vi "Barcode test.vi"() -> ()   [LabVIEW 2019]
uses:
  LLB/Commonly VI/Main Glb.vi
  LLB/Commonly VI.lvlib
  Ctrl/MeasureDisplayTab.ctl
panel:
  in  "AddTable for S2":string[][](table)=[["PCBA BARCODE", ""], ["硬體(Tool初始化)", ""], ["company(Tool初始化)", ""], ["耗電流 uA(電流表)", "T"], ["電池負載電壓", "T"], ["晶片ID(Tool FORMAT)", "F"], ["雷雕ID(TOOl scan、藍芽接收器)", "S"], ["Format(Tool FORMAT)", "F"], ["Programe(Tool Programe)", "P"]]
  out "output array":string[][](array[string])
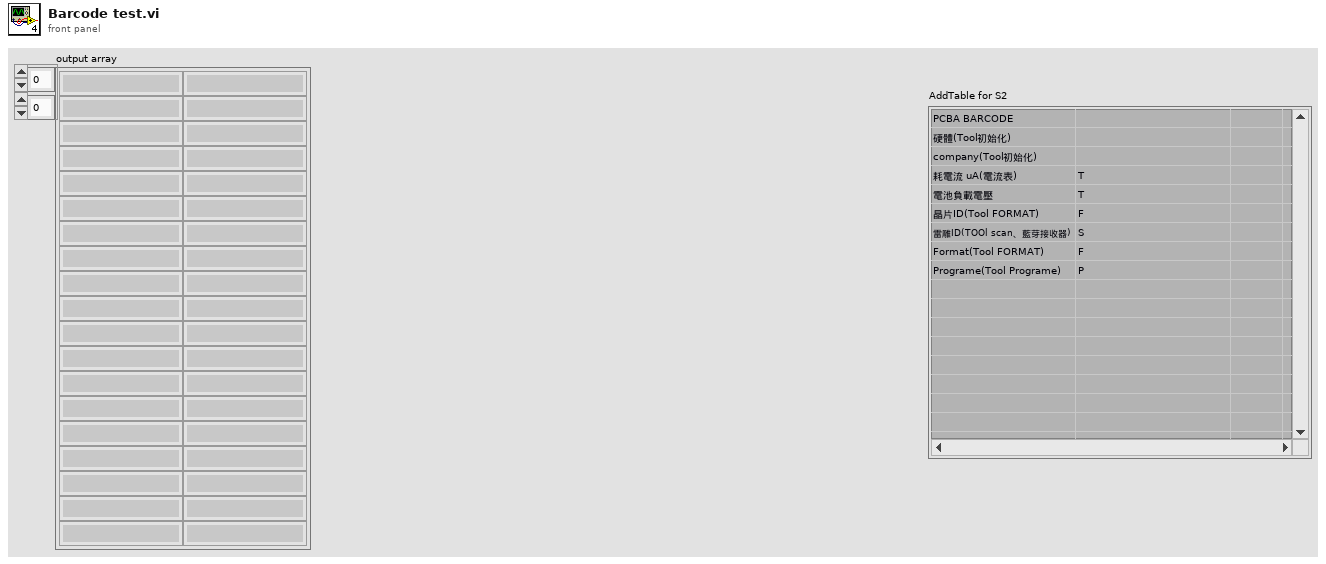
[diagram p1: front panel]
types:
  T1 = enum16{"initial", "Add", "Write", "Replace", "Delete", "REad"}
  T2 = typedef "MeasureDisplayTab.ctl" = enum16{"Tray Barcode", "PCBA BARCODE", "硬體(Tool初始化)", "company(Tool初始化)", "耗電流 uA(電流表)", "電池負載電壓", "晶片ID(Tool FORMAT)", "雷雕ID(TOOl scan、藍芽接收器)", "Format(Tool FORMAT)", "Programe(Tool Programe)", "MAC(藍芽接收器)", "ID(藍芽接收器)", "KPA(藍芽接收器)", "溫度(藍芽接收器)", "SENSOR電池電壓(藍芽接收器)", "RSSI(藍芽接收器)", "SensorType_315(FSK scan)", "FSKsnVol_315(FSK scan)", "FSKscanl_315(FSK scan)", "P_315(FSK scan)", "T_315(FSK scan)", "SensorType_433(ASK scan)", "ASKsnVol_433(ASK scan)", "ASKscan_433(ASK scan)", "P_433(ASK scan)", "T_433(ASK scan)", "測高Data"}
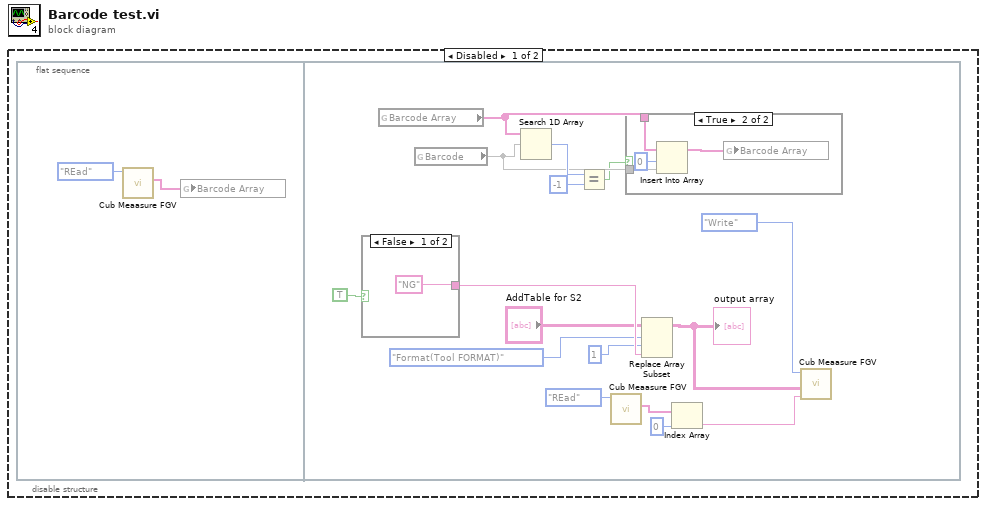
[diagram p0: block diagram]
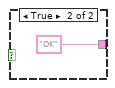
[diagram p2: hidden frame]
diagram:
  n1 = disable-structure shown="Disabled" {
    frame Disabled {
      n2 = flat-sequence {
        frame #0 {
          n3 = call "Cub Meaasure FGV.vi"("Enum"=T1."REad") -> ("Barcode Array"=w1:string[])  [unwired: 9 in, 1 out]
          n4 = global write "Main Glb.vi" "Barcode Array"(w1) -> ()
        }
        frame #1 {
          n5 = case shown="False" TRUE {
            tunnel: ["NG" "OK"] -> w7
            frame False {
            }
            frame True {
            }
          }
          n6 = global read "Main Glb.vi" "Barcode Array"() -> (w16:string[])
          n7 = global read "Main Glb.vi" "Barcode"() -> (w15)
          n8 = Search 1D Array(1D array=w16, element=w15) -> (index of element=w18:i32)  [unwired: 1 in]
          n9 = Equal?(x=w18, y=-1) -> (x = y?=w14:bool)
          n10 = call "Cub Meaasure FGV.vi"("Enum"=T1."REad") -> ("Barcode Array"=w11:string[])  [unwired: 9 in, 1 out]
          n11 = case shown="True" w14 {
            tunnel: w16 -> [_ w24]
            tunnel: w15 -> [_ w23]
            frame False {
            }
            frame True {
              n12 = Insert Into Array(array=w24, index=0, new element=w23) -> (w21:string[])
              n13 = global write "Main Glb.vi" "Barcode Array"(w21) -> ()
            }
          }
          n14 = Replace Array Subset(array="AddTable for S2", new element=w7, index (row)=MeasureDisplayTab."Format(Tool FORMAT)", index (col)=1) -> (w9:string[][])
          "output array" <- w9
          n15 = Index Array(array=w11, index=0) -> (element=w13:string)
          n16 = call "Cub Meaasure FGV.vi"("SN"=w13, "WriteTable"=w9, "Enum"=T1."Write") -> ()  [unwired: 7 in, 2 out]
        }
      }
    }
    frame Enabled {
    }
  }
